vi "06-字符串.vi"() -> ()   [LabVIEW 2025]
panel:
  out "转化后的数字":dbl
  in  "数字字符串":string
  out "连接的字符串2":string
  out "连接的字符串":string
  out "length":i32
  in  "String":string
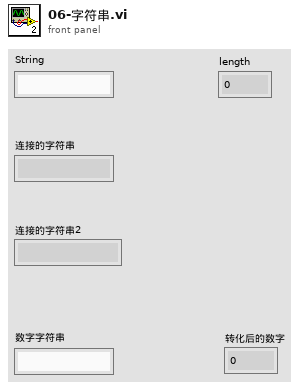
[diagram p1: front panel]
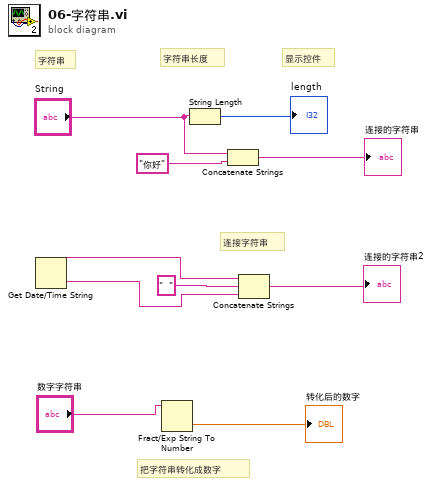
[diagram p0: block diagram]
diagram:
  # "把字符串转化成数字"
  # "连接字符串"
  # "显示控件"
  # "字符串长度"
  # "字符串"
  n1 = Get Date/Time String() -> (date string=w6:string, time string=w3:string)  [unwired: 3 in]
  n2 = Fract/Exp String To Number(string="数字字符串") -> (number=→"转化后的数字":dbl)  [unwired: 3 in, 1 out]
  n3 = String Length(string="String") -> (length=→"length":i32)
  n4 = Concatenate Strings("String", "你好" ("concatenated string")) -> (→"连接的字符串":string)
  n5 = Concatenate Strings(w6, "  " ("string"), w3) -> (→"连接的字符串2":string)
